vi "Better Steer Angle V2.vi"(5 "Current Angle":dbl(knob)=41.7137932364482 scale=0.0..360.0, 6 "Current Position":dbl, 7 "Set Point In":dbl) -> (0 "Better Angle":dbl(knob)=41.7137932364482 scale=0.0..360.0, 1 "Better Position":dbl, 2 "Encoder Count to Move":dbl, 3 "Flip motors?":bool, 4 "Degres To Travel":dbl)   [LabVIEW 2020]
uses:
  <vilib>/Analysis/coordinate.llb/Angle Range (Degree).ctl
  <vilib>/Analysis/coordinate.llb/Angle Units.ctl
  <vilib>/Analysis/coordinate.llb/Wrap Angle (scalar).vi
  <vilib>/Analysis/NI_AAL_Angle.lvlib
panel:
  out "Set Point":dbl(knob)=41.7137932364482 scale=0.0..360.0
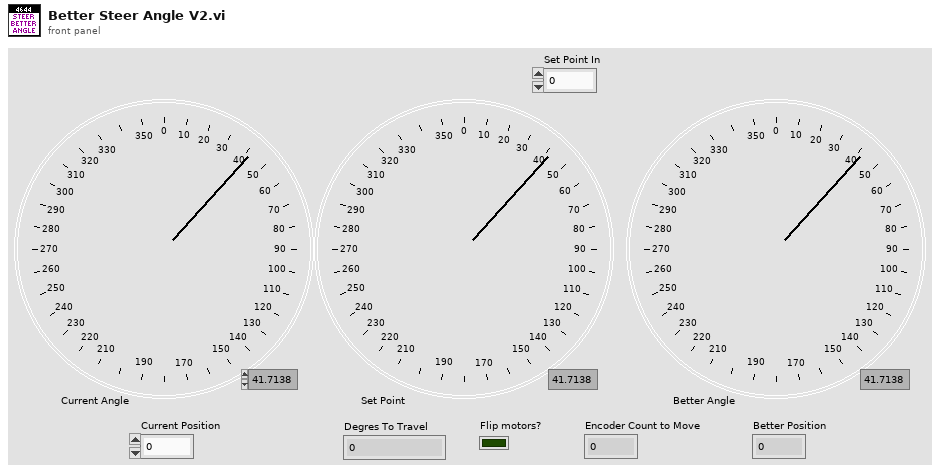
[diagram p1: front panel]
types:
  T1 = typedef "NI_AAL_Angle.lvlib/Angle Range (Degree).ctl" = u16
  T2 = typedef "NI_AAL_Angle.lvlib/Angle Units.ctl" = i32
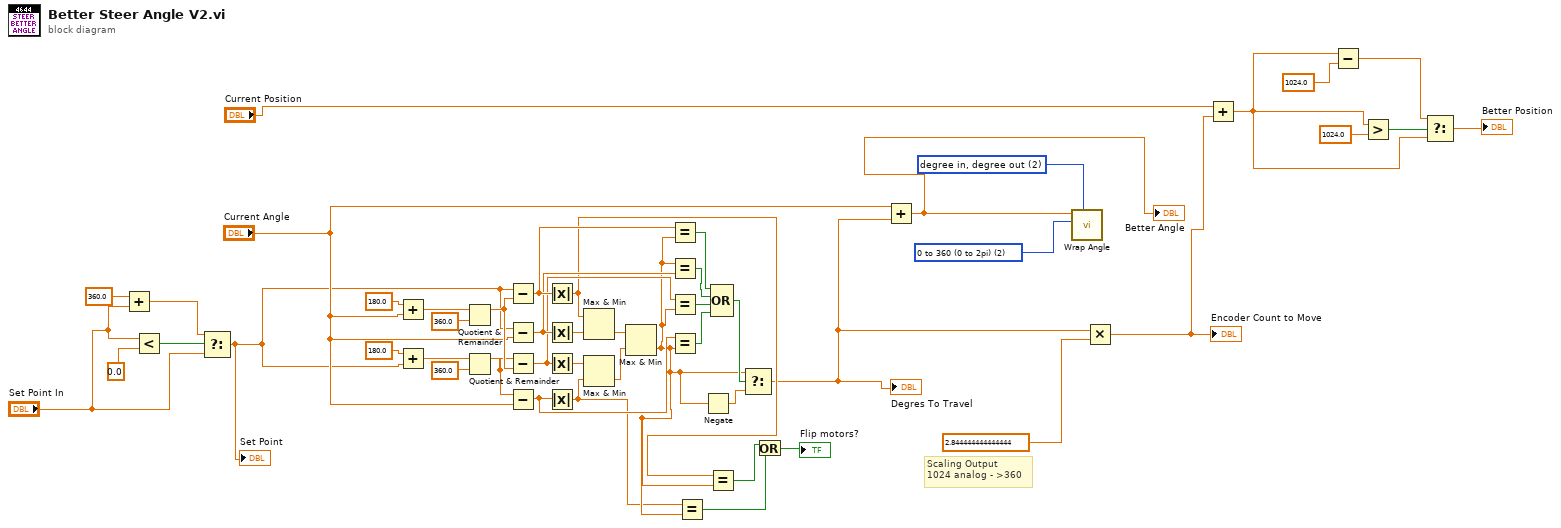
[diagram p0: block diagram]
diagram:
  w19 = T1 2 items=["none", "-180 to 180 (-pi to pi)", "0 to 360 (0 to 2pi)"] ("angle range")
  w20 = T2 2 items=["radian in, radian out", "radian in, degree out", "degree in, degree out", "degree in, radian out"] ("angle units")
  # "Scaling Output\n1024 analog - >360"
  n1 = Add(x=360.0, y="Set Point In") -> (x+y=w3:dbl)
  n2 = Less?(x="Set Point In", y=0.0) -> (x < y?=w5:bool)
  n3 = Select(t=w3, s=w5, f="Set Point In") -> (s? t:f=w1:dbl)
  "Set Point" <- w1
  n4 = Add(x=180.0, y="Current Angle") -> (x+y=w43:dbl)
  n5 = Add(x=180.0, y=w1) -> (x+y=w46:dbl)
  n6 = Quotient & Remainder(x=w43, y=360.0) -> (x-y*floor(x/y)=w42:dbl)  [unwired: 1 out]
  n7 = Quotient & Remainder(x=w46, y=360.0) -> (x-y*floor(x/y)=w36:dbl)  [unwired: 1 out]
  n8 = Subtract(x=w1, y=w42) -> (x-y=w31:dbl)
  n9 = Subtract(x=w1, y="Current Angle") -> (x-y=w30:dbl)
  n10 = Subtract(x=w36, y=w42) -> (x-y=w29:dbl)
  n11 = Subtract(x=w36, y="Current Angle") -> (x-y=w28:dbl)
  n12 = Absolute Value(x=w31) -> (abs(x)=w24:dbl)
  n13 = Absolute Value(x=w30) -> (abs(x)=w23:dbl)
  n14 = Absolute Value(x=w29) -> (abs(x)=w22:dbl)
  n15 = Absolute Value(x=w28) -> (abs(x)=w21:dbl)
  n16 = Max & Min(x=w24, y=w23) -> (min(x,y)=w40:dbl)  [unwired: 1 out]
  n17 = Max & Min(x=w22, y=w21) -> (min(x,y)=w41:dbl)  [unwired: 1 out]
  n18 = Max & Min(x=w40, y=w41) -> (min(x,y)=w27:dbl)  [unwired: 1 out]
  n19 = Equal?(x=w31, y=w27) -> (x = y?=w32:bool)
  n20 = Equal?(x=w27, y=w30) -> (x = y?=w37:bool)
  n21 = Equal?(x=w29, y=w27) -> (x = y?=w35:bool)
  n22 = Equal?(x=w28, y=w27) -> (x = y?=w33:bool)
  n23 = Equal?(x=w21, y=w27) -> (x = y?=w25:bool)
  n24 = Negate(x=w27) -> (-x=w38:dbl)
  n25 = Equal?(x=w24, y=w27) -> (x = y?=w26:bool)
  n26 = Compound Arithmetic op=OR(w32, w37, w35, w33) -> (w39:bool)
  n27 = Select(t=w27, s=w39, f=w38) -> (s? t:f=w18:dbl)
  "Degres To Travel" <- w18
  n28 = Or(x=w26, y=w25) -> (x .or. y?=→"Flip motors?":bool)
  n29 = Add(x="Current Angle", y=w18) -> (x+y=w16:dbl)
  "Better Angle" <- w16
  n30 = call-poly <vilib>:"Wrap Angle.vi"("angle units"=w20, "angle range"=w19, "angle in"=w16) -> ()  [unwired: 7 in, 2 out]
  n31 = Multiply(x=w18, y=2.844444444444444) -> (x*y=w14:dbl)
  "Encoder Count to Move" <- w14
  n32 = Add(x="Current Position", y=w14) -> (x+y=w7:dbl)
  n33 = Subtract(x=w7, y=1024.0) -> (x-y=w9:dbl)
  n34 = Greater?(x=w7, y=1024.0) -> (0:w11:bool)
  n35 = Select(t=w9, s=w11, f=w7) -> (s? t:f=→"Better Position":dbl)
